vi "Wait and Read from Oscilloscope (Manual).vi"(8 "error in (no error)":errorcluster, 9 "Collect Data":bool, 10 "data format":string, 11 "VISA resource name":refnum<visa-resource-name>) -> (0 "error out 2":errorcluster, 2 "output waveform 2":waveform(dbl)(graph), 3 "VISA resource name 2":refnum<visa-resource-name>)   [LabVIEW 2018]
doc: "Use this template to build a VI to use as a subVI."
panel:
  out "dt":dbl
  out "length 2":i32
  out "read buffer 3":string
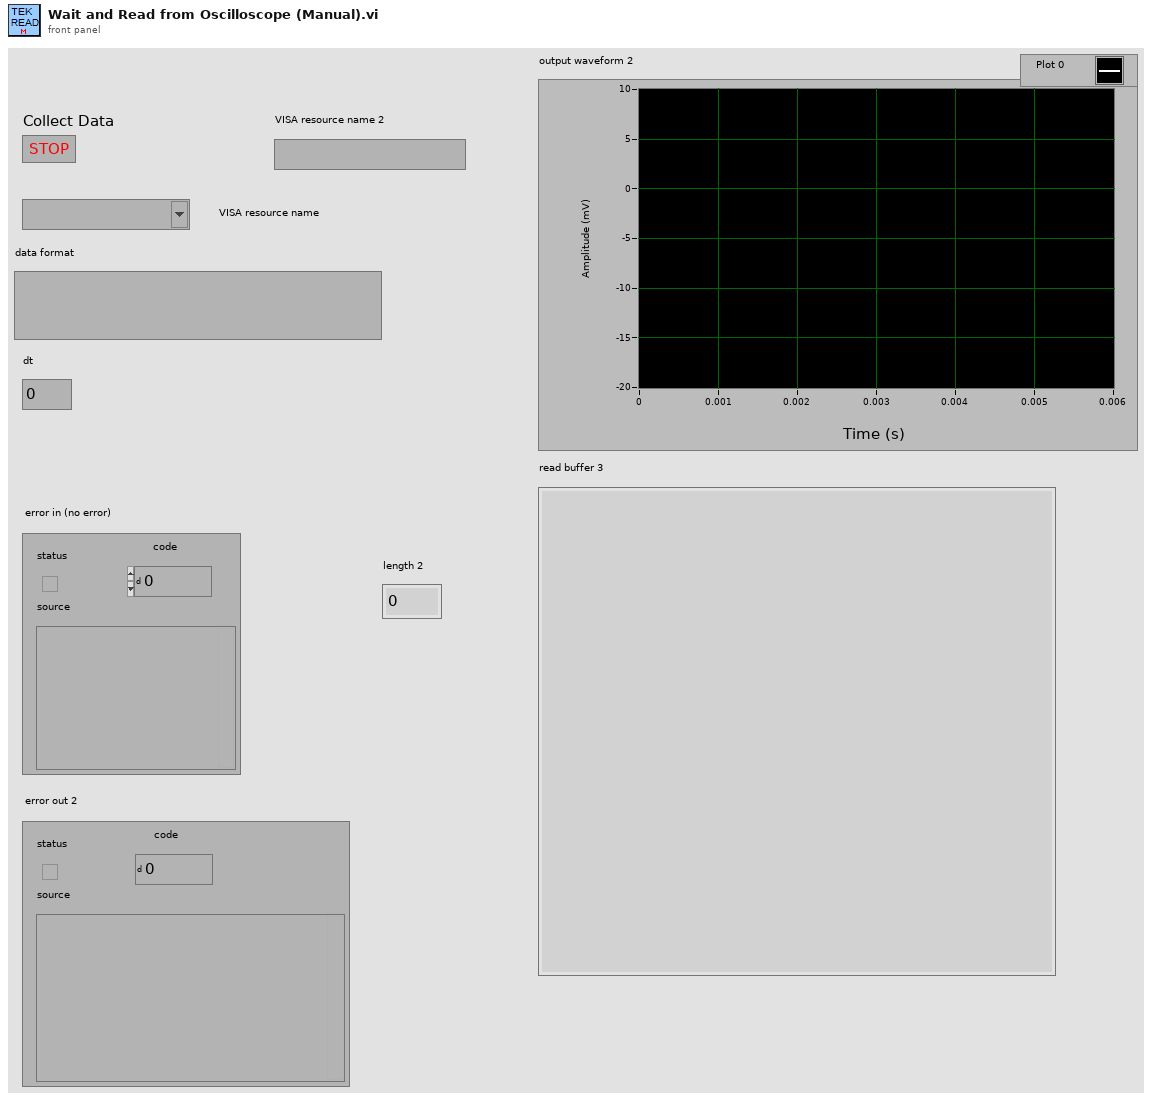
[diagram p1: front panel]
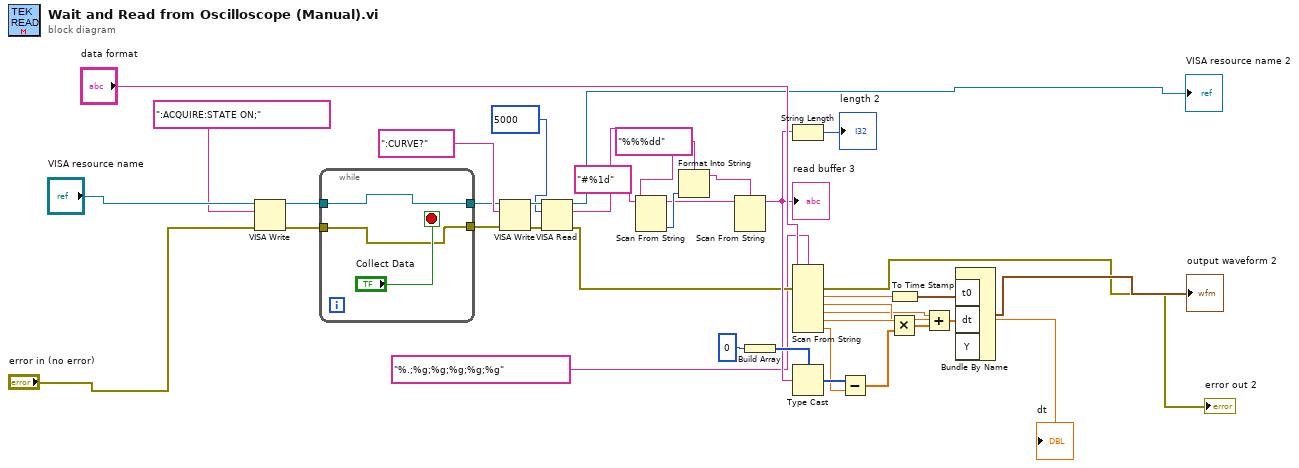
[diagram p0: block diagram]
diagram:
  n1 = VISA Write(VISA resource name="VISA resource name", write buffer=":ACQUIRE:STATE ON;", error in (no error)="error in (no error)") -> (VISA resource name out=w4:refnum<visa-resource-name>, error out=w2:errorcluster)  [unwired: 1 out]
  n2 = while {
    tunnel: w4 -> [w39]
    tunnel: [w39] -> w3
    tunnel: w2 -> [w38]
    tunnel: [w38] -> w1
    stop <- "Collect Data" stop-if-true
  }
  n3 = VISA Write(VISA resource name=w3, write buffer=":CURVE?", error in (no error)=w1) -> (VISA resource name out=w15:refnum<visa-resource-name>, error out=w16:errorcluster)  [unwired: 1 out]
  n4 = VISA Read(VISA resource name=w15, byte count=u32 5000, error in (no error)=w16) -> (VISA resource name out=→"VISA resource name 2":refnum<visa-resource-name>, read buffer=w21:string, error out=w22:errorcluster)  [unwired: 1 out]
  n5 = Scan From String(format string="#%1d", input string=w21) -> (remaining string=w9:string, output 1=w19:i32)  [unwired: 3 in, 2 out]
  n6 = Format Into String(format string="%%%dd", w19) -> (resulting string=w10:string)  [unwired: 2 in, 1 out]
  n7 = Scan From String(format string=w10, input string=w9) -> (remaining string=w29:string)  [unwired: 4 in, 2 out]
  "read buffer 3" <- w29
  n8 = Build Array(i16 0) -> (w30:i16[])
  n9 = String Length(string=w29) -> (length=→"length 2":i32)
  n10 = Scan From String(format string="%.;%g;%g;%g;%g;%g", input string="data format", error in=w22) -> (error out=→"error out 2":errorcluster, output 1=w11:dbl, output 2=w6:dbl, output 3=w5:dbl, output 4=w7:dbl, output 5=w8:dbl)  [unwired: 6 in, 2 out]
  "dt" <- w6
  n11 = Type Cast(type=w30, x=w29) -> (*(type *) &x=w28:i16[])
  n12 = Subtract(x=w28, y=w8) -> (x-y=w27:dbl[])
  n13 = Multiply(x=w7, y=w27) -> (x*y=w26:dbl[])
  n14 = To Time Stamp(1:w11) -> (0:w25:timestamp)
  n15 = Add(x=w5, y=w26) -> (x+y=w24:dbl[])
  n16 = Bundle By Name("t0"=w25, "dt"=w6, "Y"=w24) -> (→"output waveform 2":waveform(dbl))  [unwired: 1 in]
